vi "Skyline Send Waveform File.vi"(8 "error in":errorcluster, 9 "properties":cluster{"Key":string, "Value":string}[](array[cluster]) caption="properties (null)", 11 "data in":waveform(dbl)[](array[waveform])) -> (0 "error out":errorcluster, 2 "size in bytes":i32)   [LabVIEW 2017, in "Logger.lvclass"]
uses:
  logger/Logger.lvclass
  <vilib>/Skyline/File/File/Send Buffer.vi
  <vilib>/Skyline/File/File/NI Skyline File.lvclass
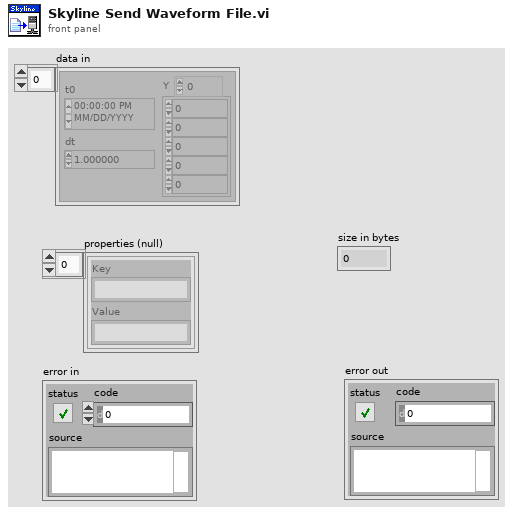
[diagram p1: front panel]
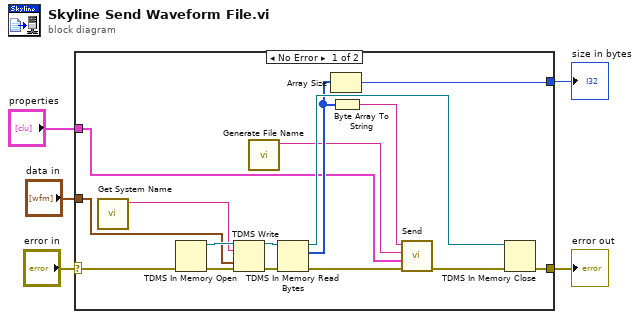
[diagram p0: block diagram]
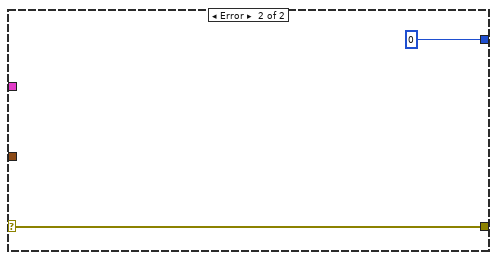
[diagram p2: hidden frame]
diagram:
  n1 = case shown="No Error" "error in" {
    selector: "error in" -> [w14 w23]
    tunnel: [w16 w23] -> w5
    tunnel: "properties" -> [w10 _]
    tunnel: "data in" -> [w20 _]
    tunnel: [w12 0] -> w1
    frame No Error {
      n2 = call "Get System Name.vi"() -> ("name"=w11:string)  [unwired: 11 in]
      n3 = TDMS In Memory Open(8:w14) -> (0:w15:errorcluster, 3:w21:refnum<k34>)  [unwired: 1 in]
      n4 = TDMS Write(0:w21, 5:w11, 9:w20, 11:w15) -> (4:w18:refnum<k34>, 15:w19:errorcluster)  [unwired: 2 in, 2 out]
      n5 = call "Generate File Name.vi"() -> ("file name"=w8:string)  [unwired: 11 in]
      n6 = TDMS In Memory Read Bytes(8:w19, 11:w18) -> (0:w9:errorcluster, 2:w13:u8[], 3:w17:refnum<k34>)  [unwired: 2 in]
      n7 = Array Size(array=w13) -> (size(s)=w12:i32)
      n8 = Byte Array To String(unsigned byte array=w13) -> (string=w7:string)
      n9 = call-poly <vilib>:"Send.vi"("error in (no error)"=w9, "properties"=w10, "file name"=w8, "data"=w7) -> ("error out"=w6:errorcluster)  [unwired: 5 in, 1 out]
      n10 = TDMS In Memory Close(8:w6, 11:w17) -> (0:w16:errorcluster)  [unwired: 2 in]
    }
    frame Error {
    }
  }
  "error out" <- w5
  "size in bytes" <- w1
